vi "TestSystem(Main).vi"() -> ()   [LabVIEW 2010]
panel:
  out "error out":errorcluster
  in  "stop":bool
  # "1. Right click and select controls\n2. Select Numeric control\n3. Move the MAIN window, see how the control inside moves \"with\" the top level vi\n4. Move the control itself\n5. Right click on control and exit\n6. Close the MAIN VI"
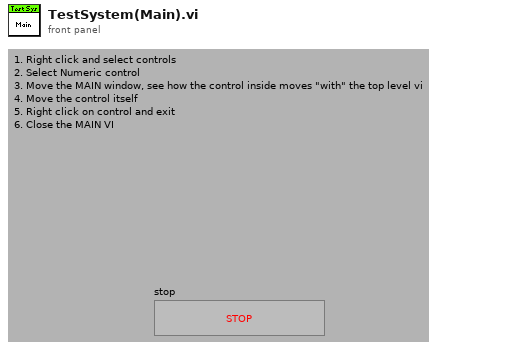
[diagram p1: front panel]
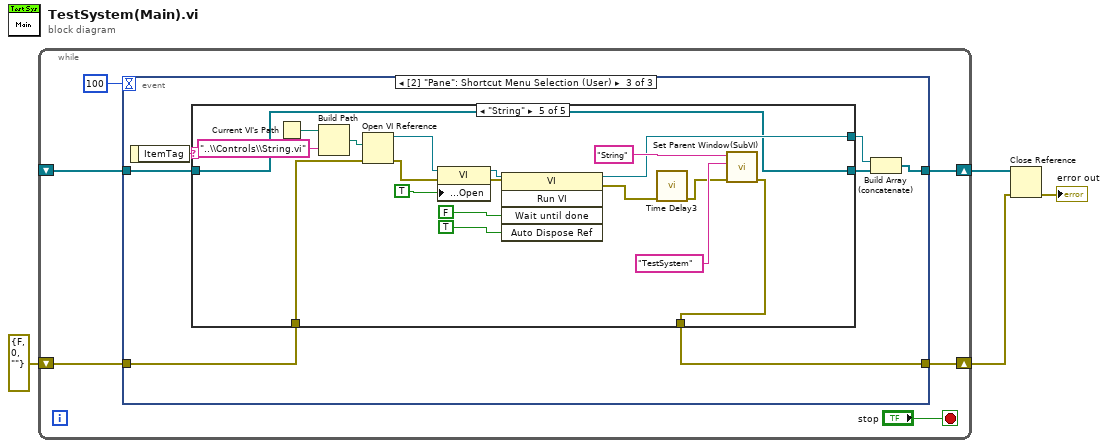
[diagram p0: block diagram]
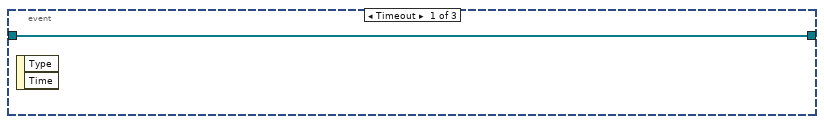
[diagram p2: hidden frame]
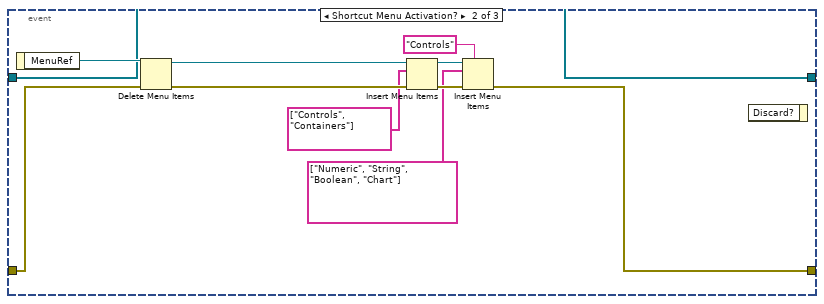
[diagram p3: hidden frame]
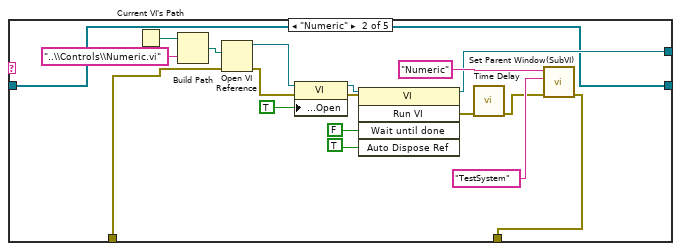
[diagram p5: hidden frame]
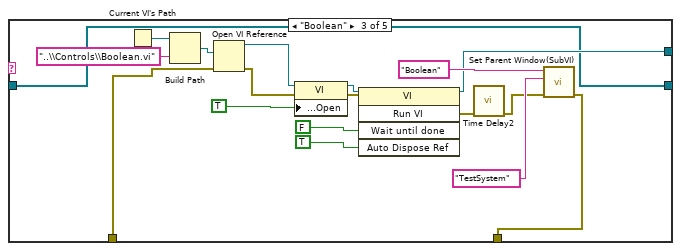
[diagram p6: hidden frame]
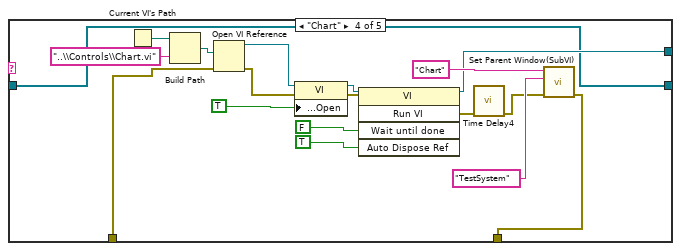
[diagram p7: hidden frame]
diagram:
  n1 = while {
    shift-right: [w8] -> w3
    shift-left: errorcluster {"status"=FALSE, "code"=0, "source"=""} ("error out") -> [w7]
    shift-right: [w5] -> w4
    shift-left: _ -> [w6]
    stop <- "stop" stop-if-true
    n2 = event shown="[2] \"Pane\": Shortcut Menu Selection (User)" {
      selector: _ -> [_ _ _]
      dyn-events: _ -> [_ _ _]
      timeout: 100 -> [_ _ _]
      tunnel: [_ w12 w27] -> w8
      tunnel: w7 -> [_ w14 w26]
      tunnel: w6 -> [w11 w13 w28]
      tunnel: [w11 w13 w23] -> w5
      event Timeout {
        n3 = event-data() -> ()  [unwired: 1 in, 2 out]
      }
      event Shortcut Menu Activation? {
        n4 = event-data() -> ("MenuRef"=w20:refnum<k9>)  [unwired: 1 in]
        n5 = Delete Menu Items(6:w14, 9:w20) -> (0:w22:errorcluster, 3:w21:refnum<k9>)  [unwired: 2 in]
        n6 = Insert Menu Items(6:w22, 8:string[] ["Controls", "Containers"], 9:w21) -> (0:w19:errorcluster, 3:w18:refnum<k9>)  [unwired: 3 in, 1 out]
        n7 = Insert Menu Items(5:"Controls" ("menu tag"), 6:w19, 8:string[] ["Numeric", "String", "Boolean", "Chart"], 9:w18) -> (0:w12:errorcluster)  [unwired: 2 in, 2 out]
        n8 = event-data() -> ()  [unwired: 2 in, 1 out]
      }
      event Shortcut Menu Selection (User) {
        n9 = event-data() -> ("ItemTag"=w29:string)  [unwired: 1 in]
        n10 = case shown="\"String\"" w29 {
          tunnel: w28 -> [w31 w38 w56 w74 w89]
          tunnel: [w31 w38 w56 w74 w89] -> w25
          tunnel: [w30 w45 w63 w81 w99] -> w27
          tunnel: w26 -> [w30 w34 w52 w70 w93]
          tunnel: [_ w39 w57 w75 w90] -> w24
          frame Default {
          }
          frame "Numeric" {
            n11 = Current VI's Path() -> (path=w36:path)
            n12 = Build Path(base path=w36, name or relative path="..\\Controls\\Numeric.vi") -> (appended path=w37:path)
            n13 = Open VI Reference(vi path=w37, error in (no error)=w34) -> (vi reference=w32:refnum<vi>, error out=w33:errorcluster)  [unwired: 4 in]
            n14 = property class="VI"(reference=w32, error in=w33, "Front Panel.Open"=TRUE ("Front Panel Window:Open")) -> (reference out=w44:refnum<vi>, error out=w43:errorcluster)
            n15 = invoke class="VI" method="Run VI"(reference=w44, error in=w43, "Wait until done"=FALSE ("Wait Until Done"), "Auto Dispose Ref"=TRUE ("Auto Dispose Reference")) -> (reference out=w39:refnum<vi>, error out=w42:errorcluster)  [unwired: 1 in, 3 out]
            n16 = call "Time Delay"("error in (no error)"=w42) -> ("error out"=w46:errorcluster)  [unwired: 10 in]
            n17 = call "Set Parent Window(SubVI).vi"("error in (no error)"=w46, "Parent Name"="TestSystem", "Child Name"="Numeric") -> ("error out"=w45:errorcluster)  [unwired: 7 in, 1 out]
          }
          frame "Boolean" {
            n18 = Current VI's Path() -> (path=w54:path)
            n19 = Build Path(base path=w54, name or relative path="..\\Controls\\Boolean.vi") -> (appended path=w55:path)
            n20 = Open VI Reference(vi path=w55, error in (no error)=w52) -> (vi reference=w50:refnum<vi>, error out=w51:errorcluster)  [unwired: 4 in]
            n21 = property class="VI"(reference=w50, error in=w51, "Front Panel.Open"=TRUE ("Front Panel Window:Open")) -> (reference out=w62:refnum<vi>, error out=w61:errorcluster)
            n22 = invoke class="VI" method="Run VI"(reference=w62, error in=w61, "Wait until done"=FALSE ("Wait Until Done"), "Auto Dispose Ref"=TRUE ("Auto Dispose Reference")) -> (reference out=w57:refnum<vi>, error out=w60:errorcluster)  [unwired: 1 in, 3 out]
            n23 = call "Time Delay2"("error in (no error)"=w60) -> ("error out"=w64:errorcluster)  [unwired: 10 in]
            n24 = call "Set Parent Window(SubVI).vi"("error in (no error)"=w64, "Parent Name"="TestSystem", "Child Name"="Boolean") -> ("error out"=w63:errorcluster)  [unwired: 7 in, 1 out]
          }
          frame "Chart" {
            n25 = Current VI's Path() -> (path=w72:path)
            n26 = Build Path(base path=w72, name or relative path="..\\Controls\\Chart.vi") -> (appended path=w73:path)
            n27 = Open VI Reference(vi path=w73, error in (no error)=w70) -> (vi reference=w68:refnum<vi>, error out=w69:errorcluster)  [unwired: 4 in]
            n28 = property class="VI"(reference=w68, error in=w69, "Front Panel.Open"=TRUE ("Front Panel Window:Open")) -> (reference out=w80:refnum<vi>, error out=w79:errorcluster)
            n29 = invoke class="VI" method="Run VI"(reference=w80, error in=w79, "Wait until done"=FALSE ("Wait Until Done"), "Auto Dispose Ref"=TRUE ("Auto Dispose Reference")) -> (reference out=w75:refnum<vi>, error out=w78:errorcluster)  [unwired: 1 in, 3 out]
            n30 = call "Time Delay4"("error in (no error)"=w78) -> ("error out"=w82:errorcluster)  [unwired: 10 in]
            n31 = call "Set Parent Window(SubVI).vi"("error in (no error)"=w82, "Parent Name"="TestSystem", "Child Name"="Chart") -> ("error out"=w81:errorcluster)  [unwired: 7 in, 1 out]
          }
          frame "String" {
            n32 = Current VI's Path() -> (path=w87:path)
            n33 = Build Path(base path=w87, name or relative path="..\\Controls\\String.vi") -> (appended path=w88:path)
            n34 = Open VI Reference(vi path=w88, error in (no error)=w93) -> (vi reference=w91:refnum<vi>, error out=w92:errorcluster)  [unwired: 4 in]
            n35 = property class="VI"(reference=w91, error in=w92, "Front Panel.Open"=TRUE ("Front Panel Window:Open")) -> (reference out=w98:refnum<vi>, error out=w97:errorcluster)
            n36 = invoke class="VI" method="Run VI"(reference=w98, error in=w97, "Wait until done"=FALSE ("Wait Until Done"), "Auto Dispose Ref"=TRUE ("Auto Dispose Reference")) -> (reference out=w90:refnum<vi>, error out=w96:errorcluster)  [unwired: 1 in, 3 out]
            n37 = call "Time Delay3"("error in (no error)"=w96) -> ("error out"=w100:errorcluster)  [unwired: 10 in]
            n38 = call "Set Parent Window(SubVI).vi"("error in (no error)"=w100, "Parent Name"="TestSystem", "Child Name"="String") -> ("error out"=w99:errorcluster)  [unwired: 7 in, 1 out]
          }
        }
        n39 = Build Array (concatenate)(w24, w25) -> (w23:refnum<vi>[])
      }
    }
  }
  n40 = Close Reference(reference=w4, error in (no error)=w3) -> (error out=→"error out":errorcluster)
